vi "Flock_Shared_FGVDebugStatus.vi"(7 "State":enum16{"Get", "Set"}(ring), 10 "DebugBoolean":bool) -> (2 "Debug Boolean":bool)   [LabVIEW 2014, in "Flock_Shared_Messaging.lvlib"]
uses:
  Flock_Shared_Messaging.lvlib
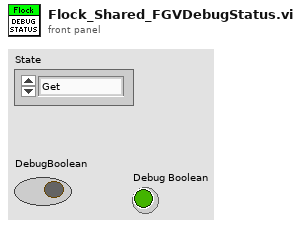
[diagram p1: front panel]
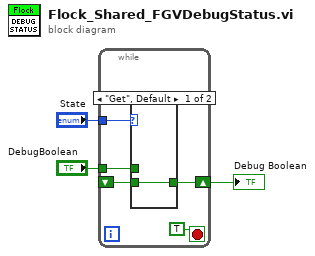
[diagram p0: block diagram]
diagram:
  n1 = while {
    tunnel: "State" -> [w7]
    tunnel: "DebugBoolean" -> [w6]
    shift-right: [w5] -> w1
    shift-left: _ -> [w4]
    stop <- TRUE stop-if-true
    n2 = case shown="\"Get\", Default" w7 {
      tunnel: w6 -> [_ w10]
      tunnel: [w9 w10] -> w5
      tunnel: w4 -> [w9 _]
      frame "Get", Default {
      }
      frame "Set" {
      }
    }
  }
  "Debug Boolean" <- w1
